vi "After Launch Init Core.vi"(8 "error in (no error)":errorcluster, 11 "CS++PVProxy in":refnum<class "CS++PVProxy.lvclass">) -> (0 "error out":errorcluster, 3 "CS++PVProxy out":refnum<class "CS++PVProxy.lvclass">)   [LabVIEW 2014, in "CS++PVProxy.lvlib" / "CS++PVProxy.lvclass"]
doc: "Use <b>Pre Launch init.vi</b> method only for sanity checks that are supposed to prevent the actor from launching if they fail. Use <B>this</B> method instead to initialize unique resources that must be released during the <b>Stop Core.vi</b> method. A corresponding high priority message will become dispatched before the <B>Actor Framework.lvlib:Actor.lvclass.Actor Core.vi</b> is called.\n\n<b>Derived classed should call the parent methode first</b> and their own initialization code after.\n\nRefer also to the ongoing discussion at https://decibel.ni.com/content/message/57394#57394."
uses:
  CS++PVProxy.lvclass
  Classes/CS++ProcessVariables/ProcessVariable/PV.lvclass
  CS++BaseActor/CS++BaseActor.lvclass/CS++BaseActor.ctl
  CS++PVProxy.lvclass/CS++PVProxy.ctl
  CS++PVMonitor Messages/CS++PVUpdate Msg/CS++PVUpdate Msg.lvclass
  CS++PVMonitor Messages/CS++PVUpdate Msg/CS++PVUpdate Msg.lvclass/CS++PVUpdate Msg.ctl
  Classes/CS++ProcessVariables/ProcessVariable/PV.lvclass/PV.ctl
  CS++PVProxy Messages/Register PVs Msg/Register PVs Msg.lvclass
  <vilib>/ActorFramework/Actor/Actor.lvclass/Actor.ctl
  <vilib>/ActorFramework/Message Enqueuer/Message Enqueuer.lvclass/Message Enqueuer.ctl
  CS++BaseActor Messages/Launch Associated GUI Msg/Launch Associated GUI Msg.lvclass/Launch Associated GUI Msg.ctl
  Classes/CS++ProcessVariables/ProcessVariable/Write Data.vi
  Classes/CS++ProcessVariables/ProcessVariable/Write Timestamp.vi
  Classes/CS++ProcessVariables/ProcessVariable/Write Quality.vi
  Classes/CS++ProcessVariables/ProcessVariable/Write status.vi
  Classes/CS++ProcessVariables/ProcessVariable/Write Type Descriptor.vi
  <vilib>/ActorFramework/Message Enqueuer/Init from Existing Queue.vi
  <vilib>/ActorFramework/Message Enqueuer/Enqueue.vi
  <vilib>/ActorFramework/Message Priority Queue/Priority Enqueue.vi
  CS++BaseActor/CS++BaseActor.lvclass
  CS++BaseActor Messages/Launch Associated GUI Msg/Launch Associated GUI Msg.lvclass
  <vilib>/ActorFramework/Message Enqueuer/Message Enqueuer.lvclass
  Classes/CS++ProcessVariables/PVConnection/PVConnection.lvclass
  Classes/CS++BaseClasses/Factory/CS++Factory.lvclass
  <vilib>/ActorFramework/Actor/Actor.lvclass
  Classes/CS++ProcessVariables/CS++ProcessVariables.lvlib
  Libraries/Utilities/CS++Utilities.lvlib
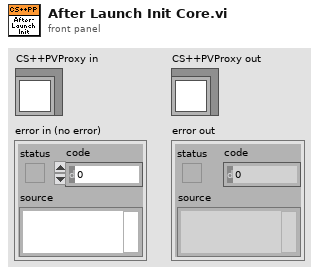
[diagram p1: front panel]
types:
  T1 = cluster{"Read Access":enum8{"Allowed", "Required", "None"}, "Write Access":enum8{"Allowed", "Required", "None"}}
  T2 = cluster{"Name":string, "Polling-String":string, "CS++PVUpdate Msg":refnum<class "CS++PVUpdate Msg.lvclass">, "PVConnection":refnum<class "PVConnection.lvclass">}[]
  T3 = cluster{"Name":string, "Polling-String":string, "CS++PVUpdate Msg out":refnum<class "CS++PVUpdate Msg.lvclass">, "PVConnection":refnum<class "PVConnection.lvclass">}
  T4 = cluster{"Name":string, "Polling-String":string, "CS++PVUpdate Msg out":refnum<class "Register PVs Msg.lvclass">, "PVConnection":refnum<class "PVConnection.lvclass">}
  T5 = cluster{"Name":string, "Polling-String":string, "CS++PVUpdate Msg out":refnum<class "CS++PVUpdate Msg.lvclass">, "PVConnection":refnum<class "PVConnection.lvclass">}[]
  T6 = cluster{"Name":string, "Polling-String":string, "CS++PVUpdate Msg":refnum<class "CS++PVUpdate Msg.lvclass">, "PVConnection":refnum<class "PVConnection.lvclass">}
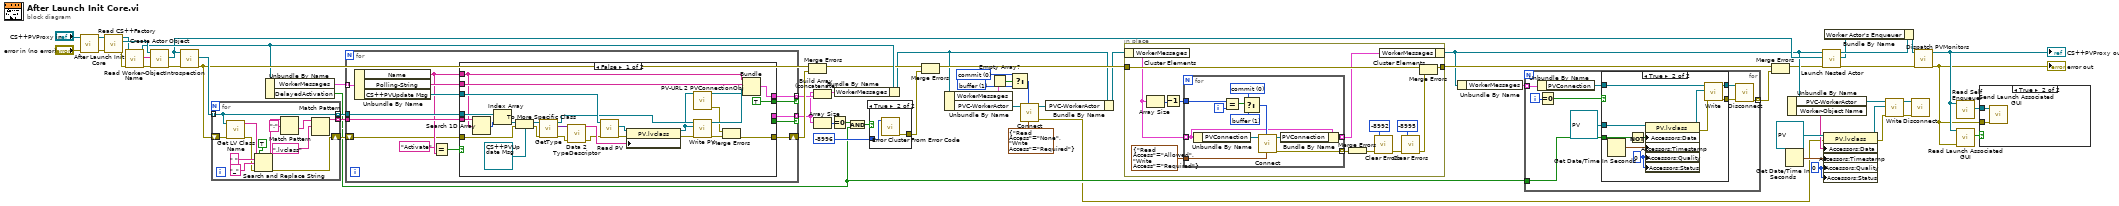
[diagram p0: block diagram]
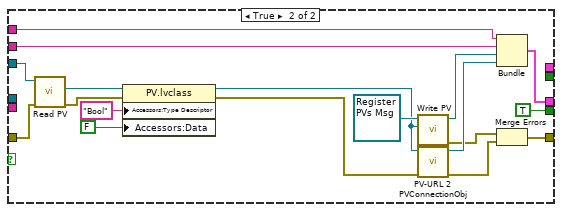
[diagram p4: hidden frame]
diagram:
  w1 = u16 1 items=["commit", "buffer"] ("Mode (buffer)")
  w2 = u16 0 items=["commit", "buffer"] ("Mode (buffer)")
  w17 = 0 ("Quality")
  n1 = call-parent "After Launch Init Core.vi"("error in (no error)"="error in (no error)", "CS++BaseActor in"="CS++PVProxy in") -> ("error out"=w32:errorcluster, "CS++BaseActor out"=w33:refnum<class "CS++PVProxy.lvclass">)  [unwired: 8 in]
  n2 = call "Read CS++Factory.vi"("error in (no error)"=w32, "CS++BaseActor in"=w33) -> ("error out"=w60:errorcluster, "CS++Factory"=w61:refnum<class "CS++Factory.lvclass">, "CS++BaseActor out"=w58:refnum<class "CS++PVProxy.lvclass">)  [unwired: 7 in]
  n3 = call-dynamic "Read Worker-Object Name.vi"("error in (no error)"=w60, "CS++PVProxy in"=w58) -> ("error out"=w59:errorcluster, "Worker-Object Name"=w57:string, "CS++PVProxy out"=w47:refnum<class "CS++PVProxy.lvclass">)  [unwired: 7 in]
  n4 = call "Create Actor Object.vi"("error in (no error)"=w59, "Object Name"=w57, "CS++Factory in"=w61) -> ("error out"=w46:errorcluster, "CS++BaseActor"=w44:refnum<class "CS++BaseActor.lvclass">)  [unwired: 5 in, 2 out]
  n5 = call "Introspection.vi"("error in (no error)"=w46, "CS++BaseActor in"=w44) -> ("error out"=w48:errorcluster, "CS++Messages"=w52:refnum<class "Message.lvclass">[])  [unwired: 7 in, 1 out]
  n6 = for {
    tunnel: w52 -> [w76] mode=indexing
    tunnel: [w76] -> w51 mode=indexing
    tunnel: [w65] -> w50 mode=indexing
    shift-right: [w69] -> w49
    shift-left: w48 -> [w75]
    n7 = call <vilib>:"Get LV Class Name.vi"("error in (no error)"=w75, "object"=w76) -> ("error out"=w70:errorcluster, "class name"=w74:string)  [unwired: 8 in]
    n8 = Search and Replace String(replace all?=TRUE ("Replace All? (false)"), input string=w74, search string=" ", replace string="_" ("Replace Pattern (\"\")"), error in=w70) -> (result string=w68:string, error out=w69:errorcluster)  [unwired: 3 in, 2 out]
    n9 = Match Pattern(string=w68, regular expression=":") -> (after substring=w66:string)  [unwired: 1 in, 3 out]
    n10 = Match Pattern(string=w66, regular expression=".lvclass") -> (before substring=w65:string)  [unwired: 1 in, 3 out]
  }
  n11 = Unbundle By Name(w47) -> ("WorkerMessages"=w53:T2, "DelayedActivation"=w23:bool)
  n12 = for {
    tunnel: w53 -> [w90] mode=indexing
    tunnel: w51 -> [w88]
    tunnel: w50 -> [w89]
    tunnel: [w81] -> w34 mode=indexing if=w82
    shift-right: [w78] -> w36
    shift-left: w49 -> [w77]
    tunnel: [w80] -> w31 mode=indexing if=w79
    n13 = Unbundle By Name(w90) -> ("Name"=w85:string, "Polling-String"=w87:string, "CS++PVUpdate Msg"=w86:refnum<class "CS++PVUpdate Msg.lvclass">)
    n14 = Equal?(x="Activate" ("regular expression"), y=w85) -> (x = y?=w83:bool)
    n15 = case shown="False" w83 {
      tunnel: w89 -> [w117 _]
      tunnel: w88 -> [w116 _]
      tunnel: w87 -> [w114 w133]
      tunnel: w77 -> [w112 w131]
      tunnel: [w104 w122] -> w78
      tunnel: w86 -> [w97 w132]
      tunnel: [w91 _] -> w81
      tunnel: w85 -> [w93 w134]
      tunnel: [TRUE _] -> w82
      tunnel: [_ w119] -> w80
      tunnel: [_ TRUE] -> w79
      frame False {
        n16 = Search 1D Array(1D array=w117, element=w93) -> (index of element=w115:i32)  [unwired: 1 in]
        n17 = Index Array(array=w116, index=w115) -> (element=w113:refnum<class "Message.lvclass">)
        n18 = To More Specific Class(target class=refnum<class "CS++PVUpdate Msg.lvclass"> refnum ("CS++PVMonitor.lvlib:CS++PVUpdate Msg.lvclass"), reference=w113, error in=w112) -> (specific class reference=w103:refnum<class "CS++PVUpdate Msg.lvclass">, error out=w102:errorcluster)
        n19 = call-dynamic "GetType.vi"("error in (no error)"=w102, "CS++PVUpdate Msg in"=w103) -> ("error out"=w98:errorcluster, "Data Sample"=w101:variant, "CS++PVUpdate Msg out"=w96:refnum<class "CS++PVUpdate Msg.lvclass">)  [unwired: 7 in]
        n20 = call "Data 2 TypeDescriptor.vi"("error in (no error)"=w98, "Data"=w101) -> ("Error Out"=w99:errorcluster, "TypeDescriptor"=w100:string)  [unwired: 8 in]
        n21 = call "Read PV.vi"("error in (no error)"=w99, "CS++PVUpdate Msg in"=w97) -> ("error out"=w109:errorcluster, "PV"=w110:refnum<class "PV.lvclass">)  [unwired: 7 in, 1 out]
        n22 = property class="PV.lvclass"(reference=w110, error in=w109, "Accessors:Type Descriptor"=w100) -> (reference out=w94:refnum<class "PV.lvclass">, error out=w108:errorcluster)
        n23 = call "PV-URL 2 PVConnectionObj.vi"("PV"=w94) -> ("Error Out"=w105:errorcluster, "PVConnection"=w107:refnum<class "PVConnection.lvclass">)  [unwired: 8 in, 1 out]
        n24 = call "Write PV.vi"("error in (no error)"=w108, "PV"=w94, "CS++PVUpdate Msg in"=w96) -> ("error out"=w106:errorcluster, "CS++PVUpdate Msg out"=w111:refnum<class "CS++PVUpdate Msg.lvclass">)  [unwired: 7 in]
        n25 = Merge Errors(w105, w106) -> (w104:errorcluster)
        n26 = Bundle("Name"=w93, "Polling-String"=w114, "CS++PVUpdate Msg out"=w111, "PVConnection"=w107) -> (w91:T3)  [unwired: 1 in]
      }
      frame True {
        n27 = call "Read PV.vi"("error in (no error)"=w131, "CS++PVUpdate Msg in"=w132) -> ("error out"=w127:errorcluster, "PV"=w128:refnum<class "PV.lvclass">)  [unwired: 7 in, 1 out]
        n28 = property class="PV.lvclass"(reference=w128, error in=w127, "Accessors:Type Descriptor"="Bool" ("Type Descriptor"), "Accessors:Data"=FALSE) -> (reference out=w126:refnum<class "PV.lvclass">, error out=w125:errorcluster)
        n29 = call "Write PV.vi"("PV"=w126, "CS++PVUpdate Msg in"=refnum<class "Register PVs Msg.lvclass"> refnum ("CS++ControllerActor.lvlib:Register PVs Msg.lvclass")) -> ("error out"=w121:errorcluster, "CS++PVUpdate Msg out"=w123:refnum<class "Register PVs Msg.lvclass">)  [unwired: 8 in]
        n30 = call "PV-URL 2 PVConnectionObj.vi"("Error In"=w125, "PV"=w126) -> ("Error Out"=w120:errorcluster, "PVConnection"=w124:refnum<class "PVConnection.lvclass">)  [unwired: 7 in, 1 out]
        n31 = Bundle("Name"=w134, "Polling-String"=w133, "CS++PVUpdate Msg out"=w123, "PVConnection"=w124) -> (w119:T4)  [unwired: 1 in]
        n32 = Merge Errors(w121, w120) -> (w122:errorcluster)
      }
    }
  }
  n33 = Merge Errors(w48, w36) -> (w29:errorcluster)
  n34 = Build Array (concatenate)(w31, w34) -> (w35:T5)
  n35 = Array Size(array=w31) -> (size(s)=w30:i32)
  n36 = Equal To 0?(x=w30) -> (x = 0?=w25:bool)
  n37 = Bundle By Name(cluster=w47, "WorkerMessages"=w35) -> (w21:refnum<class "CS++PVProxy.lvclass">)
  n38 = And(x=w25, y=w23) -> (x .and. y?=w24:bool)
  n39 = case shown="True" w24 {
    tunnel: [_ w137] -> w27
    tunnel: -8996 ("error code (0)") -> [_ w136]
    frame False {
    }
    frame True {
      n40 = call <vilib>:"Error Cluster From Error Code.vi"("error code (0)"=w136) -> ("error out"=w137:errorcluster)  [unwired: 8 in]
    }
  }
  n41 = Merge Errors(w29, w27) -> (w28:errorcluster)
  n42 = Unbundle By Name(w21) -> ("WorkerMessages"=w5:T2, "PVC-WorkerActor"=w6:refnum<class "PVConnection.lvclass">)
  n43 = Empty Array?(array=w5) -> (empty?=w4:bool)
  n44 = Select(t=w2, s=w4, f=w1) -> (s? t:f=w3:u16)
  n45 = call "Connect.vi"("Access (R/W allowed)"=T1 {"Read Access"=enum."None", "Write Access"=enum."Required"}, "Mode (buffer)"=w3, "PVConnection in"=w6) -> ("Error Out"=w9:errorcluster, "PVConnection out"=w22:refnum<class "PVConnection.lvclass">)  [unwired: 7 in]
  n46 = Bundle By Name(cluster=w21, "PVC-WorkerActor"=w22) -> (w20:refnum<class "CS++PVProxy.lvclass">)
  n47 = in-place {
    in-place-border: [w150] -> w55
    in-place-border: w28 -> [w149]
    n48 = in-place-cluster #1(w20) -> ("WorkerMessages"=w146:T2)
    n49 = Array Size(array=w146) -> (size(s)=w145:i32)
    n50 = Decrement(x=w145) -> (x-1=w144:i32)
    n51 = for {
      tunnel: w146 -> [w153] mode=indexing
      tunnel: [w152] -> w148 mode=indexing
      tunnel: T1 {"Read Access"=enum."Allowed", "Write Access"=enum."Required"} ("Access (R/W allowed)") -> [w162]
      tunnel: [w161] -> w141 mode=indexing
      tunnel: w144 -> [w159]
      i -> [w160]
      w156 = u16 1 items=["commit", "buffer"] ("Mode (commit)")
      w157 = u16 0 items=["commit", "buffer"] ("Mode (commit)")
      n52 = Unbundle By Name(w153) -> ("PVConnection"=w154:refnum<class "PVConnection.lvclass">)
      n53 = Equal?(x=w159, y=w160) -> (x = y?=w158:bool)
      n54 = Select(t=w157, s=w158, f=w156) -> (s? t:f=w155:u16)
      n55 = call "Connect.vi"("Access (R/W allowed)"=w162, "Mode (buffer)"=w155, "PVConnection in"=w154) -> ("Error Out"=w161:errorcluster, "PVConnection out"=w151:refnum<class "PVConnection.lvclass">)  [unwired: 7 in]
      n56 = Bundle By Name(cluster=w153, "PVConnection"=w151) -> (w152:T6)
    }
    n57 = Merge Errors(w141) -> (w139:errorcluster)
    n58 = call <vilib>:"Clear Errors.vi"("error in (no error)"=w139, "specific error code to clear (0: all)"=-8992) -> ("error out"=w138:errorcluster)  [unwired: 4 in, 1 out]
    n59 = in-place-cluster #1("WorkerMessages"=w148) -> (w18:refnum<class "CS++PVProxy.lvclass">)
    n60 = call <vilib>:"Clear Errors.vi"("error in (no error)"=w138, "specific error code to clear (0: all)"=-8995) -> ("error out"=w143:errorcluster)  [unwired: 4 in, 1 out]
    n61 = Merge Errors(w149, w143) -> (w150:errorcluster)
  }
  n62 = Unbundle By Name(w18) -> ("WorkerMessages"=w56:T2)
  n63 = for {
    tunnel: w56 -> [w170] mode=indexing
    tunnel: [w171] -> w54 mode=indexing
    tunnel: w23 -> [w163]
    i -> [w167]
    n64 = Unbundle By Name(w170) -> ("PVConnection"=w169:refnum<class "PVConnection.lvclass">)
    n65 = Equal To 0?(x=w167) -> (x = 0?=w164:bool)
    n66 = case shown="True" w164 {
      tunnel: w169 -> [w172 w182]
      tunnel: [w172 w181] -> w168
      tunnel: refnum<class "PV.lvclass"> refnum ("CS++ProcessVariables.lvlib:PV.lvclass") -> [_ w180]
      tunnel: [_ w177] -> w165
      tunnel: w163 -> [_ w174]
      frame False {
      }
      frame True {
        w175 = 0 ("Quality")
        n67 = Get Date/Time In Seconds() -> (seconds since 1Jan1904=w176:timestamp)
        n68 = Not(x=w174) -> (.not. x?=w173:bool)
        n69 = property class="PV.lvclass"(reference=w180, "Accessors:Data"=w173, "Accessors:Timestamp"=w176, "Accessors:Quality"=w175, "Accessors:Status"=w175) -> (reference out=w179:refnum<class "PV.lvclass">, error out=w178:errorcluster)  [unwired: 1 in]
        n70 = call "Write.vi"("error in (no error)"=w178, "PV"=w179, "PVConnection in"=w182) -> ("error out"=w177:errorcluster, "PVConnection out"=w181:refnum<class "PVConnection.lvclass">)  [unwired: 7 in]
      }
    }
    n71 = call "Disconnect.vi"("error in (no error)"=w165, "PVConnection in"=w168) -> ("error out"=w171:errorcluster)  [unwired: 8 in, 1 out]
  }
  n72 = Merge Errors(w55, w54) -> (w7:errorcluster)
  n73 = Get Date/Time In Seconds() -> (seconds since 1Jan1904=w16:timestamp)
  n74 = Unbundle By Name(w18) -> ("PVC-WorkerActor"=w13:refnum<class "PVConnection.lvclass">, "Worker-Object Name"=w14:string)
  n75 = call <vilib>:"Launch Nested Actor.vi"("error in (no error)"=w7, "Nested Actor"=w44, "Caller Actor in"=w18) -> ("error out"=w45:errorcluster, "Nested Actor's Enqueuer"=w41:refnum<class "Message Enqueuer.lvclass">, "Caller Actor out"=w43:refnum<class "CS++PVProxy.lvclass">)  [unwired: 6 in]
  n76 = property class="PV.lvclass"(reference=refnum<class "PV.lvclass"> refnum ("CS++ProcessVariables.lvlib:PV.lvclass"), error in=w9, "Accessors:Data"=w14, "Accessors:Timestamp"=w16, "Accessors:Quality"=w17, "Accessors:Status"=w17) -> (reference out=w12:refnum<class "PV.lvclass">, error out=w8:errorcluster)
  n77 = Bundle By Name(cluster=w43, "Worker Actor's Enqueuer"=w41) -> (w42:refnum<class "CS++PVProxy.lvclass">)
  n78 = call "Write.vi"("error in (no error)"=w8, "PV"=w12, "PVConnection in"=w13) -> ("error out"=w10:errorcluster, "PVConnection out"=w11:refnum<class "PVConnection.lvclass">)  [unwired: 7 in]
  n79 = call "Disconnect.vi"("error in (no error)"=w10, "PVConnection in"=w11) -> ()  [unwired: 8 in, 2 out]
  n80 = call "Dispatch PVMonitors.vi"("Error In"=w45, "CS++PVProxy in"=w42) -> ("Error Out"=w37:errorcluster, "CS++PVProxy out"=w38:refnum<class "CS++PVProxy.lvclass">)  [unwired: 8 in]
  "error out" <- w37
  "CS++PVProxy out" <- w38
  n81 = call <vilib>:"Read Self Enqueuer.vi"("Actor"=w38) -> ("Self Enqueuer"=w40:refnum<class "Message Enqueuer.lvclass">)  [unwired: 10 in]
  n82 = call "Read Launch Associated GUI.vi"("error in (no error)"=w37, "CS++BaseActor in"=w38) -> ("Launch Associated GUI"=w39:bool)  [unwired: 7 in, 2 out]
  n83 = case shown="True" w39 {
    tunnel: w40 -> [_ w184]
    tunnel: w37 -> [_ w183]
    frame False {
    }
    frame True {
      n84 = call "Send Launch Associated GUI.vi"("error in (no error)"=w183, "Message Enqueuer"=w184) -> ()  [unwired: 8 in, 2 out]
    }
  }
